vi "clear_result.vi"(8 "error in (no error)":errorcluster, 9 "clear?":bool, 11 "Plots in":refnum<class "Plots.lvclass">) -> (0 "error out":errorcluster, 3 "Plots out":refnum<class "Plots.lvclass">)   [LabVIEW 2018, in "Plots.lvclass"]
doc: "clears the results queue."
uses:
  Plots.lvclass
  Plots.lvclass/Plots.ctl
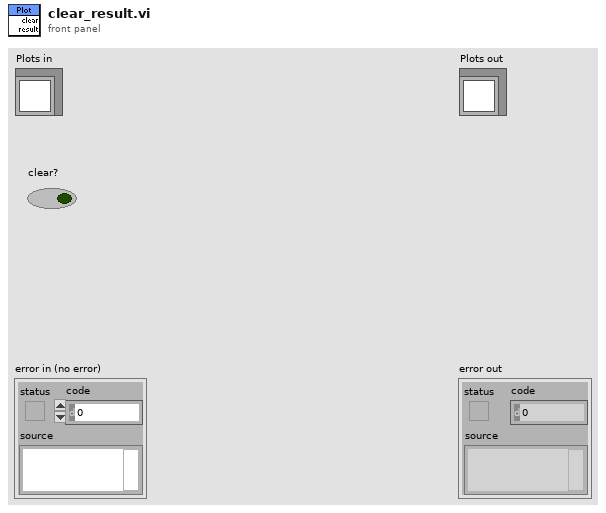
[diagram p1: front panel]
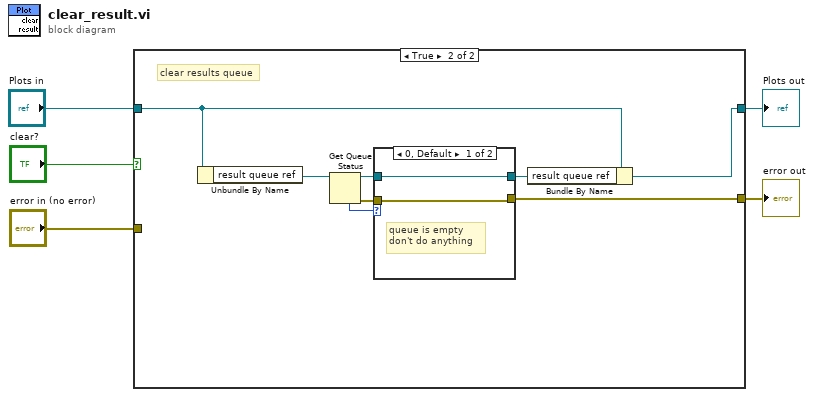
[diagram p0: block diagram]
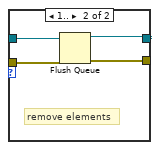
[diagram p3: hidden frame]
diagram:
  n1 = case shown="True" "clear?" {
    tunnel: [w6 w8] -> w5
    tunnel: [w7 w13] -> w3
    tunnel: "Plots in" -> [w7 w14]
    tunnel: "error in (no error)" -> [w6 _]
    frame False {
      # "don't clear results queue"
    }
    frame True {
      # "clear results queue"
      n2 = Unbundle By Name(w14) -> ("result queue ref"=w15:refnum<queue>)
      n3 = Get Queue Status(queue=w15) -> (queue out=w12:refnum<queue>, error out=w9:errorcluster, # elements in queue=w10:i32)  [unwired: 2 in, 5 out]
      n4 = case shown="0, Default" w10 {
        tunnel: w12 -> [w17 w21]
        tunnel: [w17 w19] -> w11
        tunnel: w9 -> [w16 w20]
        tunnel: [w16 w18] -> w8
        frame 0, Default {
          # "queue is empty\ndon't do anything"
        }
        frame 1.. {
          # "remove elements"
          n5 = Flush Queue(queue=w21, error in (no error)=w20) -> (queue out=w19:refnum<queue>, error out=w18:errorcluster)  [unwired: 1 out]
        }
      }
      n6 = Bundle By Name(cluster=w14, "result queue ref"=w11) -> (w13:refnum<class "Plots.lvclass">)
    }
  }
  "error out" <- w5
  "Plots out" <- w3
